vi "Configure Molbloc Position.vi"(8 "error in (no error)":errorcluster, 10 "Molbloc Position (0: A)":u16(ring) items=["A", "B", "A & B"], 11 "VISA resource name":refnum<visa-resource-name>) -> (0 "error out":errorcluster, 3 "VISA resource name out":refnum<visa-resource-name>)   [LabVIEW 2023, in "Fluke Molbox 1 Plus.lvlib"]
doc: "Selects to use the 'A', 'B' or both the 'A' and 'B' molblocs."
uses:
  Fluke Molbox 1 Plus.lvlib
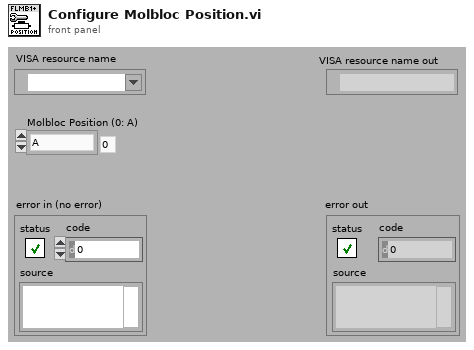
[diagram p1: front panel]
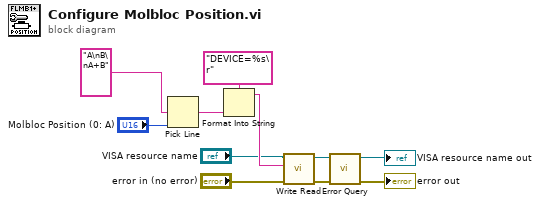
[diagram p0: block diagram]
diagram:
  n1 = Pick Line(multi-line string="A\nB\nA+B", line index="Molbloc Position (0: A)") -> (output string=w9:string)  [unwired: 1 in]
  n2 = Format Into String(format string="DEVICE=%s\r", w9) -> (resulting string=w6:string)  [unwired: 2 in, 1 out]
  n3 = call "Write Read.vi"("error in (no error)"="error in (no error)", "Write String"=w6, "VISA resource name"="VISA resource name") -> ("error out"=w3:errorcluster, "VISA resource name out"=w4:refnum<visa-resource-name>)  [unwired: 6 in, 1 out]
  n4 = call "Error Query.vi"("error in (no error)"=w3, "VISA resource name"=w4) -> ("error out"=→"error out":errorcluster, "VISA resource name out"=→"VISA resource name out":refnum<visa-resource-name>)  [unwired: 6 in, 2 out]
